vi "PicoScope6000RunBlock.vi"(7 "Acquisition Settings":T1 {"postTriggerSamples" format="%_6p"; "preTriggerSamples" format="%_6p"}, 8 "error in (no error)":errorcluster, 11 "handle in":i16) -> (0 "error out":errorcluster, 3 "handle out":i16, 4 "timeIndisposedMs":dbl, 6 "Total Requested Samples":u64)   [LabVIEW 2009]
doc: "Calls RunBlock"
uses:
  ps6000.dll
  shared/Acquisition Settings.ctl
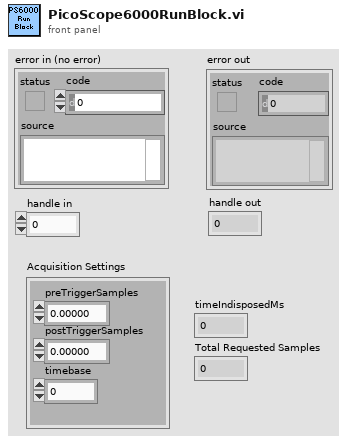
[diagram p1: front panel]
types:
  T1 = typedef "Acquisition Settings.ctl" = cluster{"preTriggerSamples":u64, "postTriggerSamples":u64, "timebase":u32}
  T2 = cluster{"status":bool, "code":u32, "source":string}
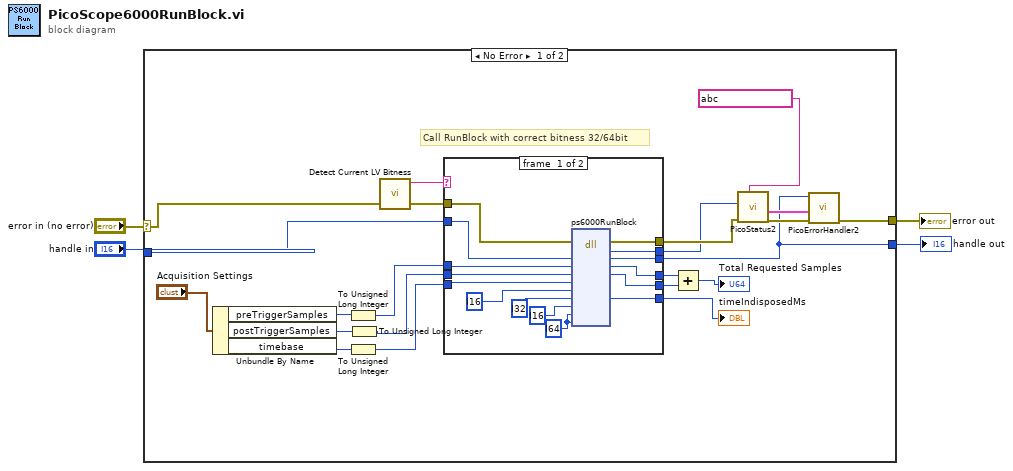
[diagram p0: block diagram]
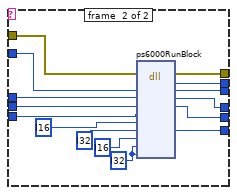
[diagram p2: hidden frame]
diagram:
  n1 = case shown="No Error" "error in (no error)" {
    selector: "error in (no error)" -> [w20 w57]
    tunnel: [w7 w57] -> w2
    tunnel: "handle in" -> [w19 w56]
    tunnel: [w5 w56] -> w3
    frame #0 {
      # "Call RunBlock with correct bitness 32/64bit"
      n2 = Unbundle By Name("Acquisition Settings") -> ("preTriggerSamples"=w23:u64, "postTriggerSamples"=w21:u64, "timebase"=w22:u32)
      n3 = To Unsigned Long Integer(number=w23) -> (unsigned 32bit integer=w17:u32)
      n4 = To Unsigned Long Integer(number=w22) -> (unsigned 32bit integer=w15:u32)
      n5 = To Unsigned Long Integer(number=w21) -> (unsigned 32bit integer=w16:u32)
      n6 = call "Detect Current LV Bitness.vi"() -> ("bitness"=w18:string)  [unwired: 11 in]
      n7 = case shown="\"32\", Default" w18 {
        tunnel: w17 -> [w40 w55]
        tunnel: [w39 w54] -> w8
        tunnel: w20 -> [w38 w53]
        tunnel: w19 -> [w37 w52]
        tunnel: w16 -> [w33 w48]
        tunnel: w15 -> [w32 w47]
        tunnel: [w30 w45] -> w14
        tunnel: [w29 w42] -> w5
        tunnel: [w28 w43] -> w13
        tunnel: [w27 w44] -> w12
        tunnel: [w26 w41] -> w6
        frame #0 {
          w35 = i64 ? ("pParameter")
          n8 = dll-call lib="PS6000.dll" fn="ps6000RunBlock" ("ps3000.dll:_ps3000_open_unit@0")(error in=w38, "handle"=w37, "preTriggerSamples"=w40, "postTriggerSamples"=w33, "timebase"=w32, "oversample"=i16 ?, "timeindisposed"=i32 ? ("pParameter"), "segmentIndex"=i16 ? ("pParameter"), "lpReady"=w35, "pParameter"=w35) -> (error out=w39:errorcluster, "PICO_STATUS"=w26:u32, "handle"=w29:i16, "preTriggerSamples"=w28:u32, "postTriggerSamples"=w27:u32, "timeindisposed"=w30:i32)  [unwired: 7 in, 1 out]
        }
        frame #1 {
          w50 = i32 ? ("pParameter")
          n9 = dll-call lib="PS6000.dll" fn="ps6000RunBlock" ("ps3000.dll:_ps3000_open_unit@0")(error in=w53, "handle"=w52, "preTriggerSamples"=w55, "postTriggerSamples"=w48, "timebase"=w47, "oversample"=i16 ?, "timeindisposed"=i32 ? ("pParameter"), "segmentIndex"=i16 ? ("pParameter"), "lpReady"=w50, "pParameter"=w50) -> (error out=w54:errorcluster, "PICO_STATUS"=w41:u32, "handle"=w42:i16, "preTriggerSamples"=w43:u32, "postTriggerSamples"=w44:u32, "timeindisposed"=w45:i32)  [unwired: 7 in, 1 out]
        }
      }
      "timeIndisposedMs" <- w14
      n10 = Add(x=w13, y=w12) -> (x+y=→"Total Requested Samples":u32)
      n11 = call "PicoStatus2.vi"("PICO source"=string ? ("source"), "Error in"=w8, "PICO STATUS"=w6) -> ("error out"=w11:errorcluster, "PICO_STATUS out"=w10:T2)  [unwired: 5 in]
      n12 = call "PicoErrorHandler2.vi"("error in (no error)"=w11, "PICO_STATUS in"=w10, "handle In"=w5) -> ("error out"=w7:errorcluster)  [unwired: 8 in]
    }
    frame #1 {
    }
  }
  "error out" <- w2
  "handle out" <- w3
